vi "Get-KeysArray-Section.vi"(8 "error in (no error)":errorcluster, 10 "Section":string, 11 "Config in":refnum<class "Config.lvclass">) -> (0 "error out":errorcluster, 2 "Array":dbl[](array[numeric]), 3 "Config out":refnum<class "Config.lvclass">)   [LabVIEW 2020]
uses:
  Config.lvclass
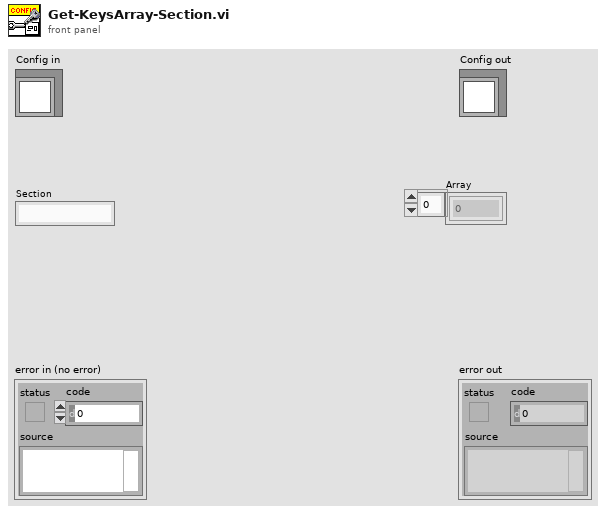
[diagram p1: front panel]
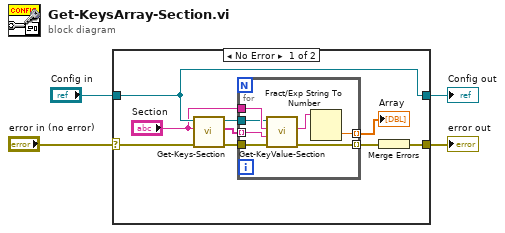
[diagram p0: block diagram]
diagram:
  n1 = case shown="No Error" "error in (no error)" {
    selector: "error in (no error)" -> [w9 w22]
    tunnel: [w7 w22] -> w3
    tunnel: [w10 w21] -> w1
    tunnel: "Config in" -> [w10 w21]
    frame No Error {
      n2 = call-dynamic "Get-Keys-Section.vi"("error in (no error)"=w9, "Section"="Section", "Config in"=w10) -> ("error out"=w12:errorcluster, "Keys"=w11:string[], "Config out"=w13:refnum<class "Config.lvclass">)  [unwired: 6 in]
      n3 = for {
        tunnel: w11 -> [w19] mode=indexing
        tunnel: w12 -> [w20]
        tunnel: "Section" -> [w18]
        tunnel: w13 -> [w17]
        tunnel: [w15] -> w6 mode=indexing
        tunnel: [w14] -> w8 mode=indexing
        n4 = call-dynamic "Get-KeyValue-Section.vi"("error in (no error)"=w20, "Key"=w19, "Section"=w18, "Config in"=w17) -> ("error out"=w14:errorcluster, "Value"=w16:string)  [unwired: 5 in, 1 out]
        n5 = Fract/Exp String To Number(string=w16) -> (number=w15:dbl)  [unwired: 3 in, 1 out]
      }
      "Array" <- w6
      n6 = Merge Errors(w8) -> (w7:errorcluster)
    }
    frame Error {
    }
  }
  "error out" <- w3
  "Config out" <- w1
